vi "4155C Output-FPP v2.0.vi"(0 "VISA resource name in":refnum<visa-resource-name>="GPIB0::14::INSTR", 1 "FPP - Source":u32(ring) items=["VSU1  ", "VSU2  "], 2 "Gate":T4={"Gate Start"=0.0, "Gate Stop"=2.0, "Gate Step"=1.0, "Gate Compliance"=0.0001, "Gate PComp"=0.0, "Range mode"=0, "Range"=6} {"Range" max=11 scale=0.0..11.0; "Range mode" items=["Auto", "Limited", "Fixed"]; "Gate PComp" format="%^.2e"; "Gate Compliance" format="%^.2e"; "Gate Step" format="%^.4e"; "Gate Stop" format="%^.4e"; "Gate Start" format="%^.4e"}, 3 "Drain":T5={"Drain Start"=0.0, "Drain Stop"=2.0, "Drain Compliance"=0.0001, "Drain Step (linear only)"=1.0, "Drain PComp"=0.0, "Range mode"=0, "Range"=6} {"Range" max=11 scale=0.0..11.0; "Range mode" items=["Auto", "Limited", "Fixed"]; "Drain PComp" format="%^.2e"; "Drain Step (linear only)" format="%^.4e"; "Drain Compliance" format="%^.2e"; "Drain Stop" format="%^.4e"; "Drain Start" format="%^.4e"}, 4 "FPP - Drain":u32(ring)=1 items=["SMU1  ", "SMU2  ", "SMU3  ", "SMU4  ", "SMU5  ", "SMU6  "], 5 "Timings":T3={"integration time"=0, "Short/Long integration time"=0.00064, "hold time (sec)"=0.0, "delay time (sec)"=0.0, "Step Time (0 disables)"=0.0, "sweep method"=0, "Pulse period"=0.005, "Base voltage"=0.0, "Pulse width"=0.0005} {"Pulse width" min=0.0005 max=0.1 step=0.0001 format="%.4f"; "Base voltage" format="%^.4e"; "Pulse period" min=0.005 max=1.0 step=0.0001 format="%.4f"; "sweep method" items=["Continuous", "Pulsed"]; "Step Time (0 disables)" format="%.2f"; "delay time (sec)" format="%.4f"; "hold time (sec)" format="%.4f"; "Short/Long integration time" format="%^.0e"; "integration time" scale=0.0..2.0}, 6 "error in (no error)":errorcluster, 8 "FPP - Gate":u32(ring)=2 items=["SMU1  ", "SMU2  ", "SMU3  ", "SMU4  ", "SMU5  ", "SMU6  "], 9 "FPP - Probe 1":u32(ring) items=["SMU1  ", "SMU2  ", "SMU3  ", "SMU4  ", "SMU5  ", "SMU6  "], 10 "sweep mode":u16(ring) items=["Single", "Double"], 11 "FPP - Probe 2":u32(ring)=3 items=["SMU1  ", "SMU2  ", "SMU3  ", "SMU4  ", "SMU5  ", "SMU6  "], 12 "Panel controls":T2={"Emergency Stop"=refnum, "OutputGraph Max"=1e-05, "Text/Graph (text=false)"=FALSE} {"OutputGraph Max" format="%.2e"}) -> (16 "VD":dbl[](array[numeric]) format="%.2f", 17 "Outparams":T1={"V2 Start"=0.0, "V2 Step"=0.0, "Number of points"=1} {"V2 Step" format="%.2f"; "V2 Start" format="%^.4e"}, 20 "VISA Resource Name out":refnum<visa-resource-name>, 21 "Vprobe2":dbl[](array[numeric]) format="%.2f", 22 "ID":dbl[](array[numeric]) format="%.2f", 23 "IG":dbl[](array[numeric]) format="%.2f", 25 "Vprobe1":dbl[](array[numeric]) format="%.2f", 26 "error out":errorcluster)   [LabVIEW 2016]
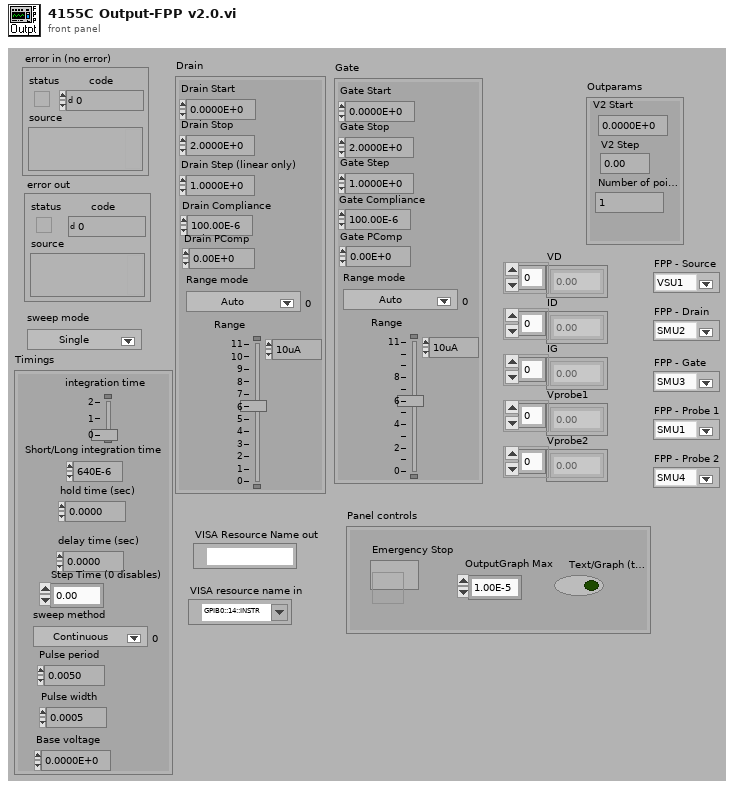
[diagram p1: front panel]
types:
  T1 = cluster{"V2 Start":dbl, "V2 Step":dbl, "Number of points":i32}
  T2 = cluster{"Emergency Stop":refnum<vi>, "OutputGraph Max":dbl, "Text/Graph (text=false)":bool}
  T3 = cluster{"integration time":u32, "Short/Long integration time":dbl, "hold time (sec)":dbl, "delay time (sec)":dbl, "Step Time (0 disables)":dbl, "sweep method":u16, "Pulse period":dbl, "Base voltage":dbl, "Pulse width":dbl}
  T4 = cluster{"Gate Start":dbl, "Gate Stop":dbl, "Gate Step":dbl, "Gate Compliance":dbl, "Gate PComp":dbl, "Range mode":u16, "Range":u8}
  T5 = cluster{"Drain Start":dbl, "Drain Stop":dbl, "Drain Compliance":dbl, "Drain Step (linear only)":dbl, "Drain PComp":dbl, "Range mode":u16, "Range":u8}
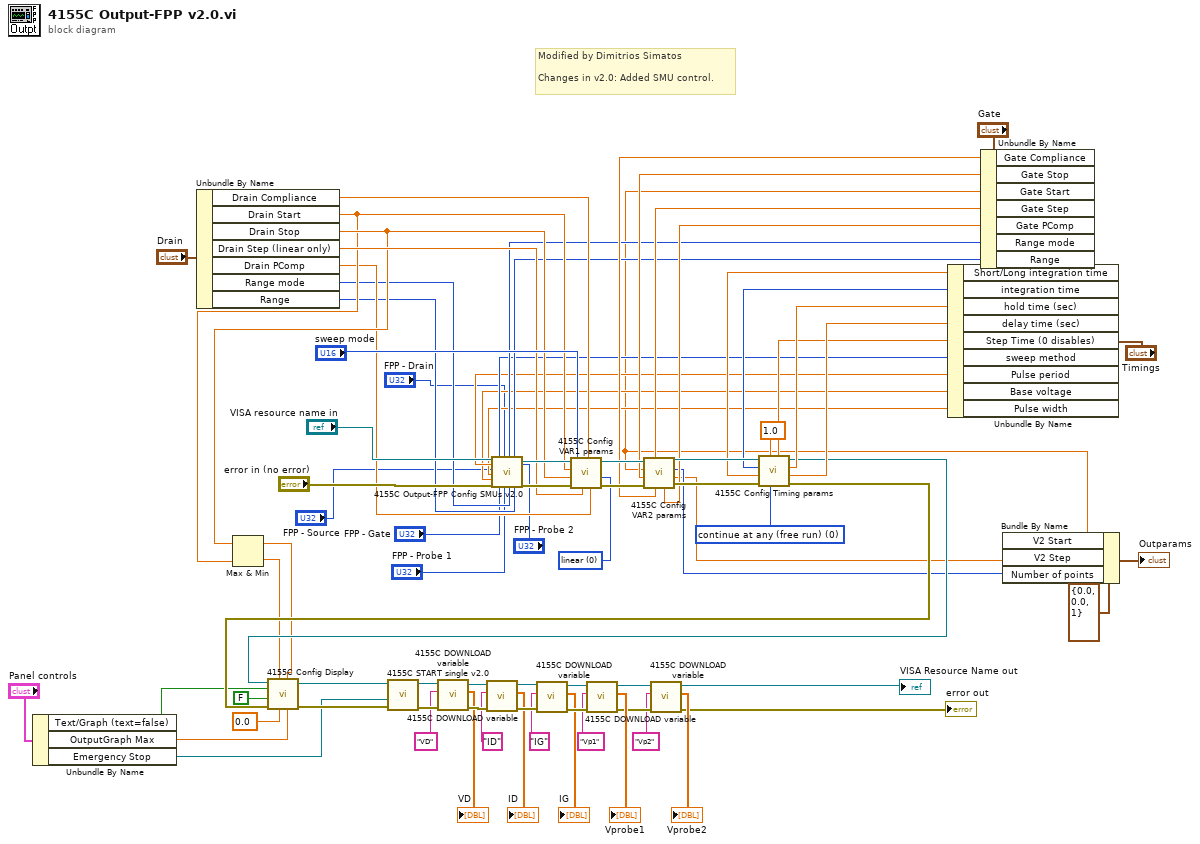
[diagram p0: block diagram]
diagram:
  w65 = u8 0 items=["continue at any (free run)", "stop at any abnorm", "stop at compliance"] ("stop condition (free run:0)")
  w62 = u16 0 items=["linear", "log 10", "log 25", "log 50"] ("sweep spacing (linear: 0)")
  # "Modified by Dimitrios Simatos\n\nChanges in v2.0: Added SMU control."
  n1 = Unbundle By Name("Panel controls") -> ("Text/Graph (text=false)"=w31:bool, "OutputGraph Max"=w30:dbl, "Emergency Stop"=w29:refnum<vi>)
  n2 = Unbundle By Name("Drain") -> ("Drain Compliance"=w49:dbl, "Drain Start"=w33:dbl, "Drain Stop"=w34:dbl, "Drain Step (linear only)"=w48:dbl, "Drain PComp"=w28:dbl, "Range mode"=w24:u16, "Range"=w23:u8)
  n3 = Max & Min(x=w34, y=w33) -> (max(x,y)=w6:dbl, min(x,y)=w7:dbl)
  n4 = Unbundle By Name("Timings") -> ("Short/Long integration time"=w67:dbl, "integration time"=w44:u32, "hold time (sec)"=w45:dbl, "delay time (sec)"=w46:dbl, "Step Time (0 disables)"=w41:dbl, "sweep method"=w22:u16, "Pulse period"=w21:dbl, "Base voltage"=w19:dbl, "Pulse width"=w20:dbl)
  n5 = Unbundle By Name("Gate") -> ("Gate Compliance"=w52:dbl, "Gate Stop"=w51:dbl, "Gate Start"=w14:dbl, "Gate Step"=w50:dbl, "Gate PComp"=w27:dbl, "Range mode"=w26:u16, "Range"=w25:u8)
  n6 = call "4155C Output-FPP Config SMUs v2.0.vi"("VISA resource name in"="VISA resource name in", "Pulse period"=w21, "FPP - Source"="FPP - Source", "Pulse width"=w20, "Base voltage"=w19, "error in (no error)"="error in (no error)", "sweep method"=w22, "FPP - Gate"="FPP - Gate", "FPP - Drain"="FPP - Drain", "FPP - Probe 1"="FPP - Probe 1", "Gate mode"=w26, "Source/drain mode"=w24, "Gate Range"=w25, "Source/drain Range"=w23, "FPP - Probe 2"="FPP - Probe 2") -> ("VISA Resource Name out"=w60:refnum<visa-resource-name>, "error out"=w59:errorcluster)  [unwired: 3 in]
  n7 = call "4155C Config VAR1 params.vi"("sweep spacing (linear: 0)"=w62, "power compliance (0 = OFF)"=w28, "compliance"=w49, "step (linear only)"=w48, "sweep mode"="sweep mode", "error in (no error)"=w59, "stop"=w34, "start"=w33, "VISA session"=w60) -> ("error out"=w63:errorcluster, "dup VISA resource name"=w64:refnum<visa-resource-name>)  [unwired: 1 out]
  n8 = call "4155C Config VAR2 params.vi"("power compliance (0 = OFF)"=w27, "compliance"=w52, "step"=w50, "error in (no error)"=w63, "stop"=w51, "start"=w14, "VISA session"=w64) -> ("error out"=w68:errorcluster, "Corrected Step"=w15:dbl, "Number of points"=w16:i32, "dup VISA resource name"=w69:refnum<visa-resource-name>)  [unwired: 1 in]
  n9 = call "4155C Config Timing params.vi"("delay time (sec)"=w46, "hold time (sec)"=w45, "Step Time (0 disables)"=w41, "stop condition (free run:0)"=w65, "wait time parameter"=1.0, "error in (no error)"=w68, "Short/Long integration time"=w67, "integration time"=w44, "VISA session"=w69) -> ("error out"=w38:errorcluster, "dup VISA resource name"=w37:refnum<visa-resource-name>)  [unwired: 1 in]
  n10 = call "4155C Config Display.vi"("Ymax"=w30, "Var1 Stop"=w6, "Ymin"=0.0, "Var1 Start"=w7, "error in (no error)"=w38, "Logarithmic"=FALSE, "SPA Display"=w31, "VISA session"=w37) -> ("error out"=w39:errorcluster, "dup VISA resource name"=w40:refnum<visa-resource-name>)  [unwired: 2 in]
  n11 = call "4155C START single v2.0.vi"("error in (no error)"=w39, "Emergency Stop"=w29, "VISA resource name in"=w40) -> ("error out"=w80:errorcluster, "VISA Resource Name out"=w81:refnum<visa-resource-name>)  [unwired: 3 in]
  n12 = call "4155C DOWNLOAD variable.vi"("error in (no error)"=w80, "Variable name"="VD", "VISA resource name in"=w81) -> ("error out"=w78:errorcluster, "Output data"=→"VD":dbl[], "VISA Resource Name out"=w77:refnum<visa-resource-name>)  [unwired: 2 in]
  n13 = call "4155C DOWNLOAD variable.vi"("error in (no error)"=w78, "Variable name"="ID", "VISA resource name in"=w77) -> ("error out"=w74:errorcluster, "Output data"=→"ID":dbl[], "VISA Resource Name out"=w75:refnum<visa-resource-name>)  [unwired: 2 in]
  n14 = call "4155C DOWNLOAD variable.vi"("error in (no error)"=w74, "Variable name"="IG", "VISA resource name in"=w75) -> ("error out"=w73:errorcluster, "Output data"=→"IG":dbl[], "VISA Resource Name out"=w72:refnum<visa-resource-name>)  [unwired: 2 in]
  n15 = call "4155C DOWNLOAD variable.vi"("error in (no error)"=w73, "Variable name"="Vp1", "VISA resource name in"=w72) -> ("error out"=w13:errorcluster, "Output data"=→"Vprobe1":dbl[], "VISA Resource Name out"=w12:refnum<visa-resource-name>)  [unwired: 2 in]
  n16 = call "4155C DOWNLOAD variable.vi"("error in (no error)"=w13, "Variable name"="Vp2", "VISA resource name in"=w12) -> ("error out"=→"error out":errorcluster, "Output data"=→"Vprobe2":dbl[], "VISA Resource Name out"=→"VISA Resource Name out":refnum<visa-resource-name>)  [unwired: 2 in]
  n17 = Bundle By Name(cluster=T1 {"V2 Start"=0.0, "V2 Step"=0.0, "Number of points"=1} ("Outparams"), "V2 Start"=w14, "V2 Step"=w15, "Number of points"=w16) -> (→"Outparams":T1)
